vi "Measurement UI.vi"() -> ()   [LabVIEW 2021, in "Linearity_DAC.lvlib"]
uses:
  Linearity_DAC.lvlib
panel:
  out "INL index":u32 caption="INL Index"
  out "DNL index":u32 caption="DNL Index"
  out "INL":dbl format="%_6g"
  out "DNL":dbl format="%_6g"
  out "DNL INL waveform":dbl[][](graph)
  out "Transfer function":T1(graph)
  in  "settings tab":enum32{"Measurement", "HiddenControls"}(tab)
  in  "Full scale range":u32=10 caption="FULL SCALE RANGE"
  in  "DMM resolution":dbl(ring)=5.5 caption="DIGITS OF RESOLUTION" items=["3.5"=3.5, "4.5"=4.5, "5.5"=5.5, "6.5"=6.5, "7.5"=7.5]
  in  "DMM range":dbl=10.0 caption="RANGE" format="%.1g"
  in  "DMM resource":string caption="DMM RESOURCE"
  in  "Sweep stop code":u32=3968 caption="SWEEP STOP CODE"
  in  "Sweep start code":u32=32 caption="SWEEP START CODE"
  in  "DAC channel":u32 caption="DAC CHANNEL"
  in  "Digital resource":string caption="DIGITAL RESOURCE"
  out "Digital codes":u32[](array[numeric])
  out "DNL waveform":dbl[](array[numeric]) format="%_6g"
  out "INL waveform":dbl[](array[numeric]) format="%_6g"
  out "DMM readings":dbl[](array[numeric]) format="%_6g"
  # "Generation settings"
  # "Acquisition settings"
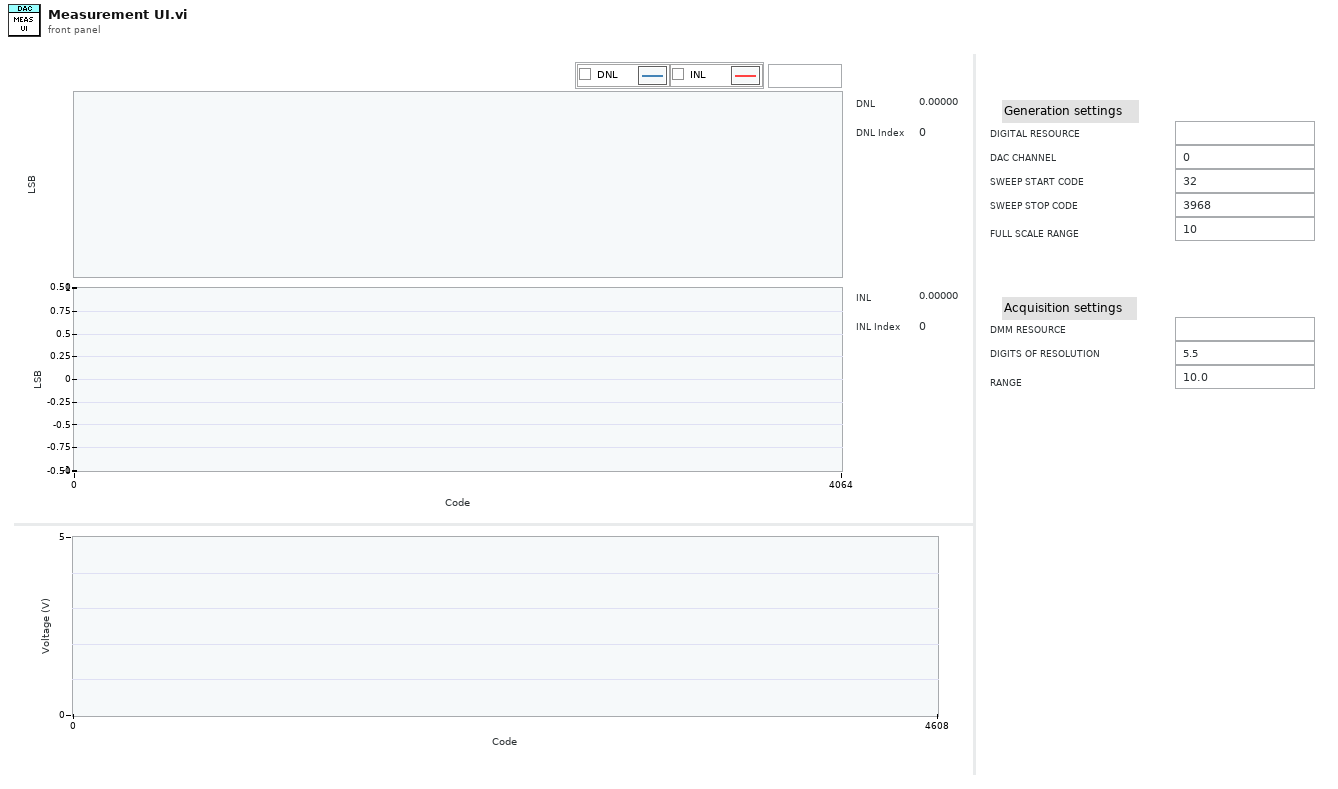
[diagram p1: front panel]
types:
  T1 = cluster{"Digital codes":u32[], "DMM readings":dbl[]}
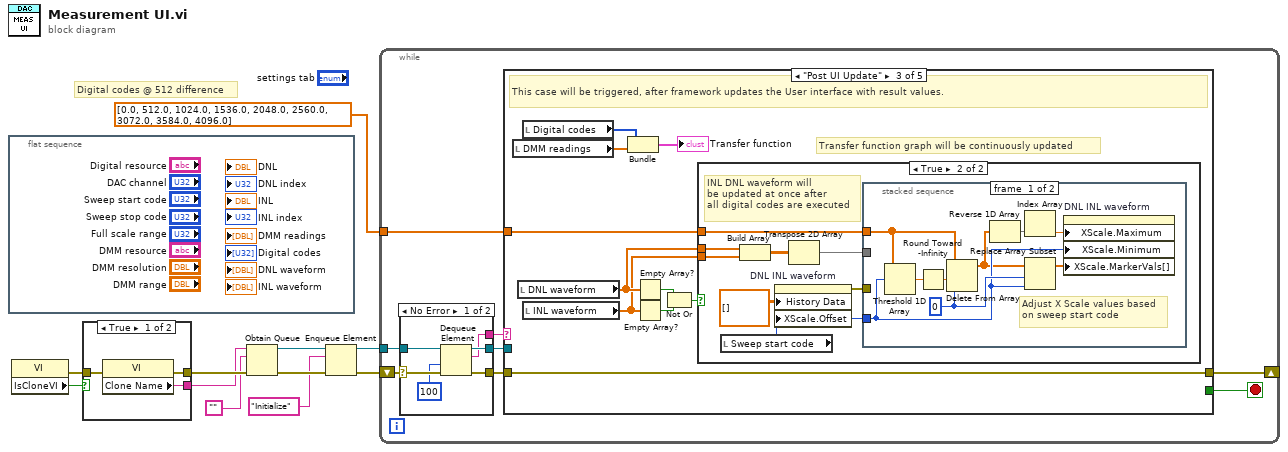
[diagram p0: block diagram]
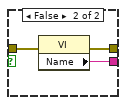
[diagram p2: hidden frame]
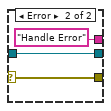
[diagram p3: hidden frame]
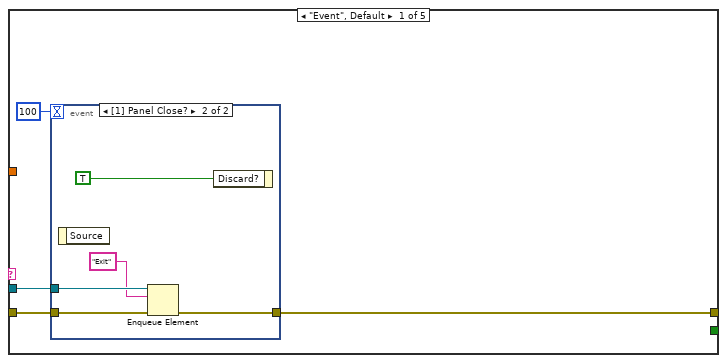
[diagram p4: hidden frame]
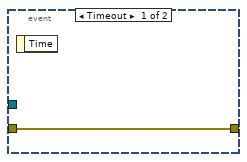
[diagram p5: hidden frame]
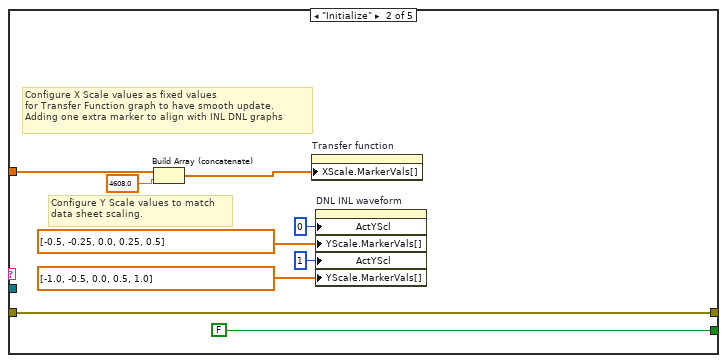
[diagram p6: hidden frame]
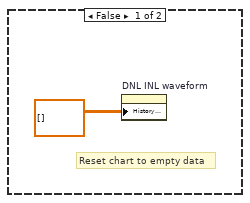
[diagram p7: hidden frame]
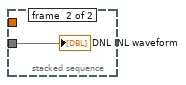
[diagram p8: hidden frame]
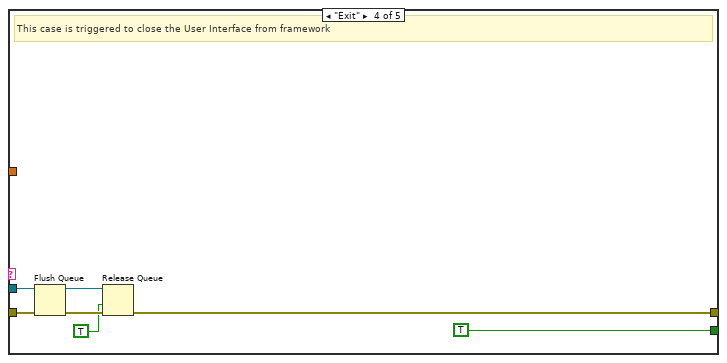
[diagram p9: hidden frame]
diagram:
  # "Digital codes @ 512 difference"
  n1 = flat-sequence {
    frame #0 {
    }
  }
  n2 = property class="VI"() -> (error out=w2:errorcluster, "IsCloneVI"=w3:bool)  [unwired: 2 in, 1 out]
  n3 = case shown="True" w3 {
    tunnel: [w14 w17] -> w11
    tunnel: [w13 w16] -> w10
    tunnel: w2 -> [w12 w15]
    frame True {
      n4 = property class="VI"(error in=w12) -> (error out=w14:errorcluster, "Clone Name"=w13:string)  [unwired: 1 in, 1 out]
    }
    frame False {
      n5 = property class="VI"(error in=w15) -> (error out=w17:errorcluster, "Name"=w16:string)  [unwired: 1 in, 1 out]
    }
  }
  n6 = Obtain Queue(name (unnamed)=w10, element data type="", error in (no error)=w11) -> (queue out=w7:refnum<queue>, error out=w9:errorcluster)  [unwired: 2 in, 1 out]
  n7 = Enqueue Element(queue=w7, element="Initialize", error in (no error)=w9) -> (queue out=w6:refnum<queue>, error out=w8:errorcluster)  [unwired: 1 in, 1 out]
  n8 = while {
    shift-right: [w20] -> _
    shift-left: w8 -> [w25]
    tunnel: w6 -> [w23]
    tunnel: dbl[] [0.0, 512.0, 1024.0, 1536.0, 2048.0, 2560.0, 3072.0, 3584.0, 4096.0] ("Y Scale.Marker Values[]") -> [w18]
    stop <- w19 stop-if-true
    n9 = case shown="No Error" w25 {
      selector: w25 -> [w31 w34]
      tunnel: [w30 w34] -> w24
      tunnel: w23 -> [w29 w33]
      tunnel: [w28 w33] -> w22
      tunnel: [w27 "Handle Error"] -> w21
      frame No Error {
        n10 = Dequeue Element(queue=w29, timeout in ms (-1)=100, error in (no error)=w31) -> (queue out=w28:refnum<queue>, element=w27:string, error out=w30:errorcluster)  [unwired: 1 out]
      }
      frame Error {
      }
    }
    n11 = case shown="\"Post UI Update\"" w21 {
      tunnel: w24 -> [w37 w53 w63 w89 w90]
      tunnel: w22 -> [w35 _ _ w87 _]
      tunnel: [w38 w53 w63 w84 w90] -> w20
      tunnel: [_ FALSE _ TRUE _] -> w19
      tunnel: w18 -> [_ w47 w54 _ _]
      frame "Event", Default {
        n12 = event shown="[1] Panel Close?" {
          selector: _ -> [_ _]
          dyn-events: _ -> [_ _]
          timeout: 100 -> [_ _]
          tunnel: [w39 w42] -> w38
          tunnel: w37 -> [w39 w43]
          tunnel: w35 -> [_ w41]
          event Timeout {
            n13 = event-data() -> ()  [unwired: 1 in, 1 out]
          }
          event Panel Close? {
            n14 = event-data() -> ()  [unwired: 1 in, 1 out]
            n15 = Enqueue Element(queue=w41, element="Exit", error in (no error)=w43) -> (error out=w42:errorcluster)  [unwired: 1 in, 2 out]
            n16 = event-data("Discard?"=TRUE) -> ()  [unwired: 1 in, 1 out]
          }
        }
      }
      frame "Initialize" {
        # "Configure Y Scale values to match\ndata sheet scaling."
        # "Configure X Scale values as fixed values \nfor Transfer Function graph to have smooth update.\nAdding one extra marker to align with INL DNL graphs"
        n17 = Build Array (concatenate)(w47, 4608.0) -> (w46:dbl[])
        n18 = property on="Transfer function" class="XYGraph (strict)"("XScale.MarkerVals[]"=w46) -> ()  [unwired: 2 in, 2 out]
        n19 = property on="DNL INL waveform" class="WFChart (strict)"("ActYScl"=0 ("Active Y Scale"), "YScale.MarkerVals[]"=dbl[] [-0.5, -0.25, 0.0, 0.25, 0.5] ("Y Scale.Marker Values[]"), "ActYScl"=1 ("Active Y Scale"), "YScale.MarkerVals[]"=dbl[] [-1.0, -0.5, 0.0, 0.5, 1.0] ("Y Scale.Marker Values[]")) -> ()  [unwired: 2 in, 2 out]
      }
      frame "Post UI Update" {
        # "Transfer function graph will be continuously updated"
        # "This case will be triggered, after framework updates the User interface with result values."
        n20 = local read "DMM readings"() -> (w61:dbl[])
        n21 = local read "DNL waveform"() -> (w56:dbl[])
        n22 = local read "Digital codes"() -> (w62:u32[])
        n23 = local read "INL waveform"() -> (w55:dbl[])
        n24 = Bundle("Digital codes"=w62, "DMM readings"=w61) -> (→"Transfer function":T1)  [unwired: 1 in]
        n25 = Empty Array?(array=w56) -> (empty?=w59:bool)
        n26 = Empty Array?(array=w55) -> (empty?=w58:bool)
        n27 = Not Or(1:w58, 2:w59) -> (0:w57:bool)
        n28 = case shown="True" w57 {
          tunnel: w56 -> [_ w70]
          tunnel: w55 -> [_ w69]
          tunnel: w54 -> [_ w66]
          frame False {
            # "Reset chart to empty data"
            n29 = property on="DNL INL waveform" class="WFChart (strict)"("History Data"=dbl[][] []) -> ()  [unwired: 2 in, 2 out]
          }
          frame True {
            # "INL DNL waveform will\nbe updated at once after\nall digital codes are executed"
            n30 = local read "Sweep start code"() -> (w65:u32)
            n31 = Build Array(w70, w69) -> (w71:dbl[][])
            n32 = property on="DNL INL waveform" class="WFChart (strict)"("History Data"=dbl[][] [], "XScale.Offset"=w65) -> (error out=w67:errorcluster)  [unwired: 2 in, 1 out]
            n33 = Transpose 2D Array(2D array=w71) -> (transposed array=w68:dbl[][])
            n34 = stacked-sequence {
              tunnel: w68 -> [_ w82]
              tunnel: w67 -> [_ _]
              tunnel: w66 -> [w76 _]
              tunnel: w65 -> [w77 _]
              frame #0 {
                w79 = 0 ("index")
                # "Adjust X Scale values based\non sweep start code"
                n35 = Threshold 1D Array(2:w77, 3:w76) -> (0:w81:dbl)  [unwired: 1 in]
                n36 = Round Toward -Infinity(1:w81) -> (0:w80:dbl)
                n37 = Delete From Array(array=w76, length=w80, index=w79) -> (array with subset deleted=w73:dbl[])  [unwired: 1 out]
                n38 = Reverse 1D Array(array=w73) -> (reversed array=w75:dbl[])
                n39 = Index Array(array=w75) -> (element=w74:dbl)  [unwired: 1 in]
                n40 = Replace Array Subset(array=w73, new element=w77, index=w79) -> (w78:dbl[])
                n41 = property on="DNL INL waveform" class="WFChart (strict)"("XScale.Maximum"=w74, "XScale.Minimum"=w77, "XScale.MarkerVals[]"=w78) -> ()  [unwired: 2 in, 2 out]
              }
              frame #1 {
                "DNL INL waveform" <- w82
              }
            }
          }
        }
      }
      frame "Exit" {
        # "This case is triggered to close the User Interface from framework"
        n42 = Flush Queue(queue=w87, error in (no error)=w89) -> (queue out=w86:refnum<queue>, error out=w85:errorcluster)  [unwired: 1 out]
        n43 = Release Queue(queue=w86, force destroy? (F)=TRUE, error in (no error)=w85) -> (error out=w84:errorcluster)  [unwired: 2 out]
      }
      frame "Handle Error" {
      }
    }
  }
